vi "to negative fixint.vi"(8 "error in":errorcluster, 11 "byte":u8=2 format="%b") -> (0 "error out":errorcluster, 3 "negative fix int":i8)   [LabVIEW 2020, in "wamplv.lvlib" / "MessagePack.lvclass"]
uses:
  MessagePack.lvclass
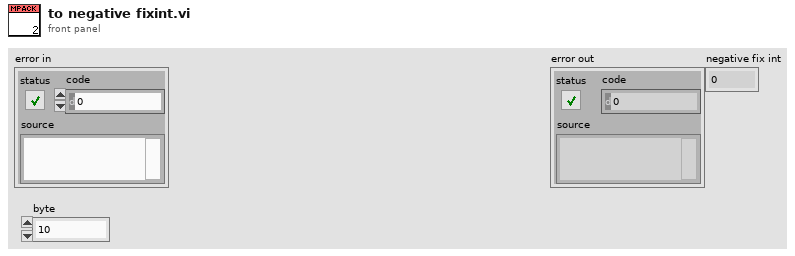
[diagram p1: front panel]
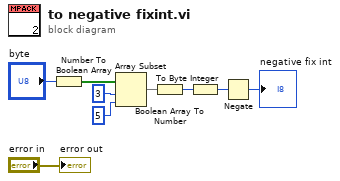
[diagram p0: block diagram]
diagram:
  n1 = Number To Boolean Array(number="byte") -> (Boolean array=w7:bool[])
  n2 = Array Subset(array=w7, index=3, length=5) -> (w4:bool[])
  n3 = Boolean Array To Number(Boolean array=w4) -> (number=w3:u32)
  n4 = To Byte Integer(number=w3) -> (8bit integer=w2:i8)
  n5 = Negate(x=w2) -> (-x=→"negative fix int":i8)
  "error out" <- "error in"
